vi "ReleaseQueueElem.vi"   [LabVIEW 2019]
uses:
  GraphsQueue.vi
  Global.lvlib
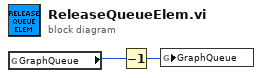
[diagram p0: block diagram]
diagram:
  n1 = global read "GraphsQueue.vi" "GraphQueue"() -> (w2:i16)
  n2 = Decrement(x=w2) -> (x-1=w1:i16)
  n3 = global write "GraphsQueue.vi" "GraphQueue"(w1) -> ()
